vi "Generate_WayPoints_Hopping_CV_AntiDrift.vi"(11 "Input Cluster":T2={"Scan Rate (um/s)"=15.0, "X Start"=15.0, "X End"=15.0, "Y Start"=15.0, "Y End"=15.0, " Z Start"=15.0, "HoppingDistance"=1.0, "V"=15.0, "Z End"=15.0, "Approach Rate Hopping (um/s)"=15.0, "Retrack Rate (um/s)"=15.0, "V 2"=15.0, "Approach Rate (um/s)"=15.0, "V 3"=15.0, "CV Rate / V/s"=15.0, "V 4"=15.0, "V 1"=15.0, "HoldTime1/s"=15.0, "Hold time 2 / s"=15.0, "Hold time 3/ s"=15.0}) -> (0 "output cluster":T1)   [LabVIEW 2023]
uses:
  TypeDefs/WayPointCluster.ctl
  User_Vi/Settings.vi
panel:
  in  "WayPointCluster":T1
  out "Y  P":dbl
  out "X  P":dbl
  out "HoppingDistanceX":dbl
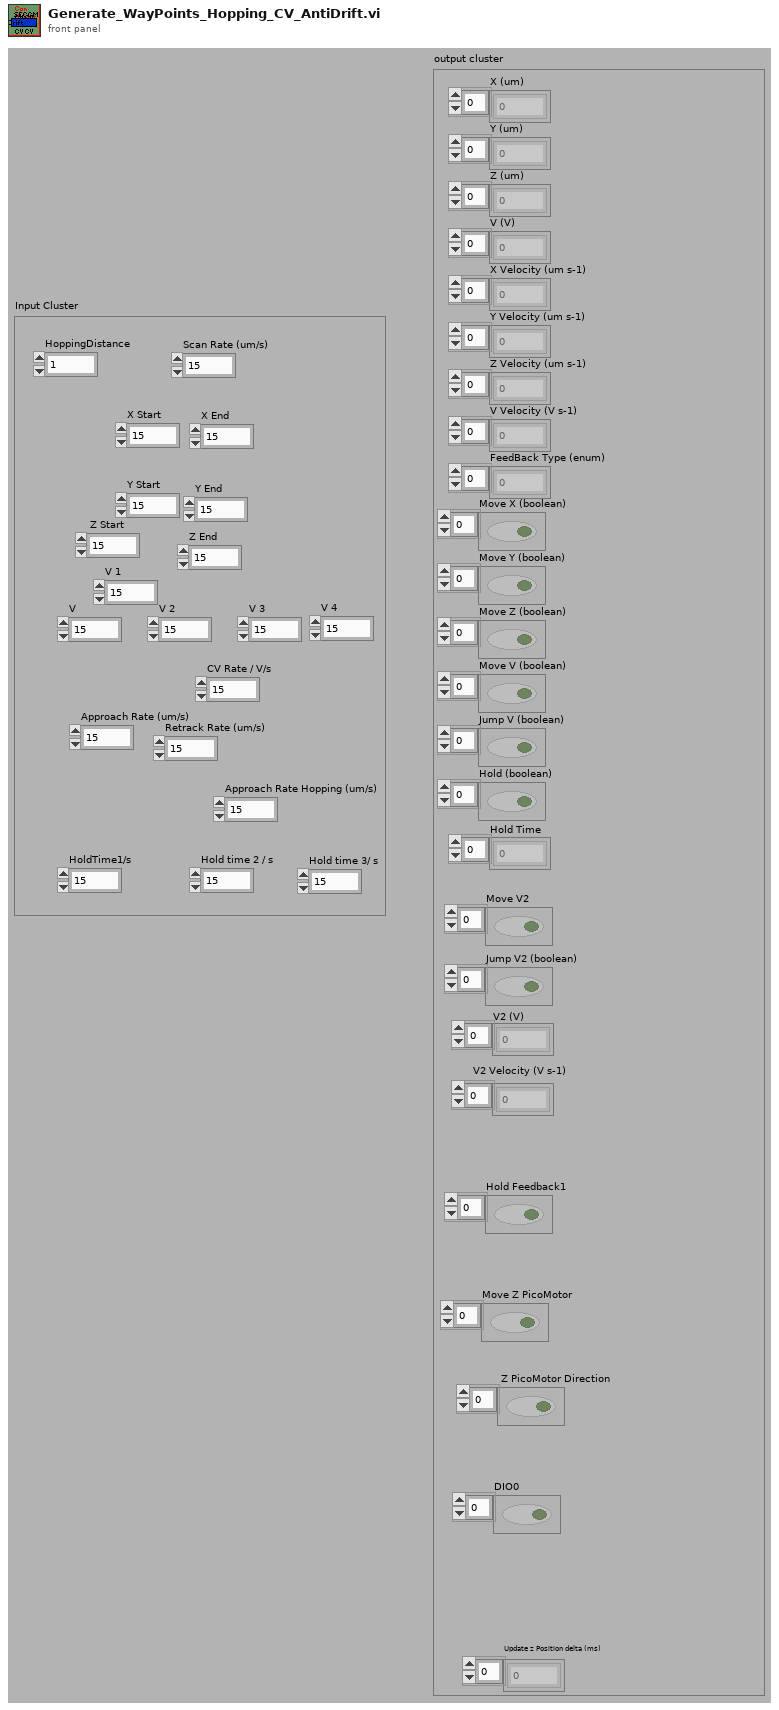
[diagram p1: front panel]
types:
  T1 = typedef "WayPointCluster.ctl" = cluster{"X (um)":dbl[], "Y (um)":dbl[], "Z (um)":dbl[], "V (V)":dbl[], "X Velocity (um s-1)":dbl[], "Y Velocity (um s-1)":dbl[], "Z Velocity (um s-1)":dbl[], "V Velocity (V s-1)":dbl[], "FeedBack Type (enum)":u16[], "Move X (boolean)":bool[], "Move Y (boolean)":bool[], "Move Z (boolean)":bool[], "Move V (boolean)":bool[], "Jump V (boolean)":bool[], "Hold (boolean)":bool[], "Hold Time":u32[], "V2 (V)":dbl[], "Move V2":bool[], "V2 Velocity (V s-1)":dbl[], "Jump V2 (boolean)":bool[], "Update z Position delta (ms)":i16[], "Hold Feedback1":bool[], "Move Z PicoMotor":bool[], " Z PicoMotor Direction":bool[], "DIO0":bool[]}
  T2 = cluster{"Scan Rate (um/s)":dbl, "X Start":dbl, "X End":dbl, "Y Start":dbl, "Y End":dbl, " Z Start":dbl, "HoppingDistance":dbl, "V":dbl, "Z End":dbl, "Approach Rate Hopping (um/s)":dbl, "Retrack Rate (um/s)":dbl, "V 2":dbl, "Approach Rate (um/s)":dbl, "V 3":dbl, "CV Rate / V/s":dbl, "V 4":dbl, "V 1":dbl, "HoldTime1/s":dbl, "Hold time 2 / s":dbl, "Hold time 3/ s":dbl}
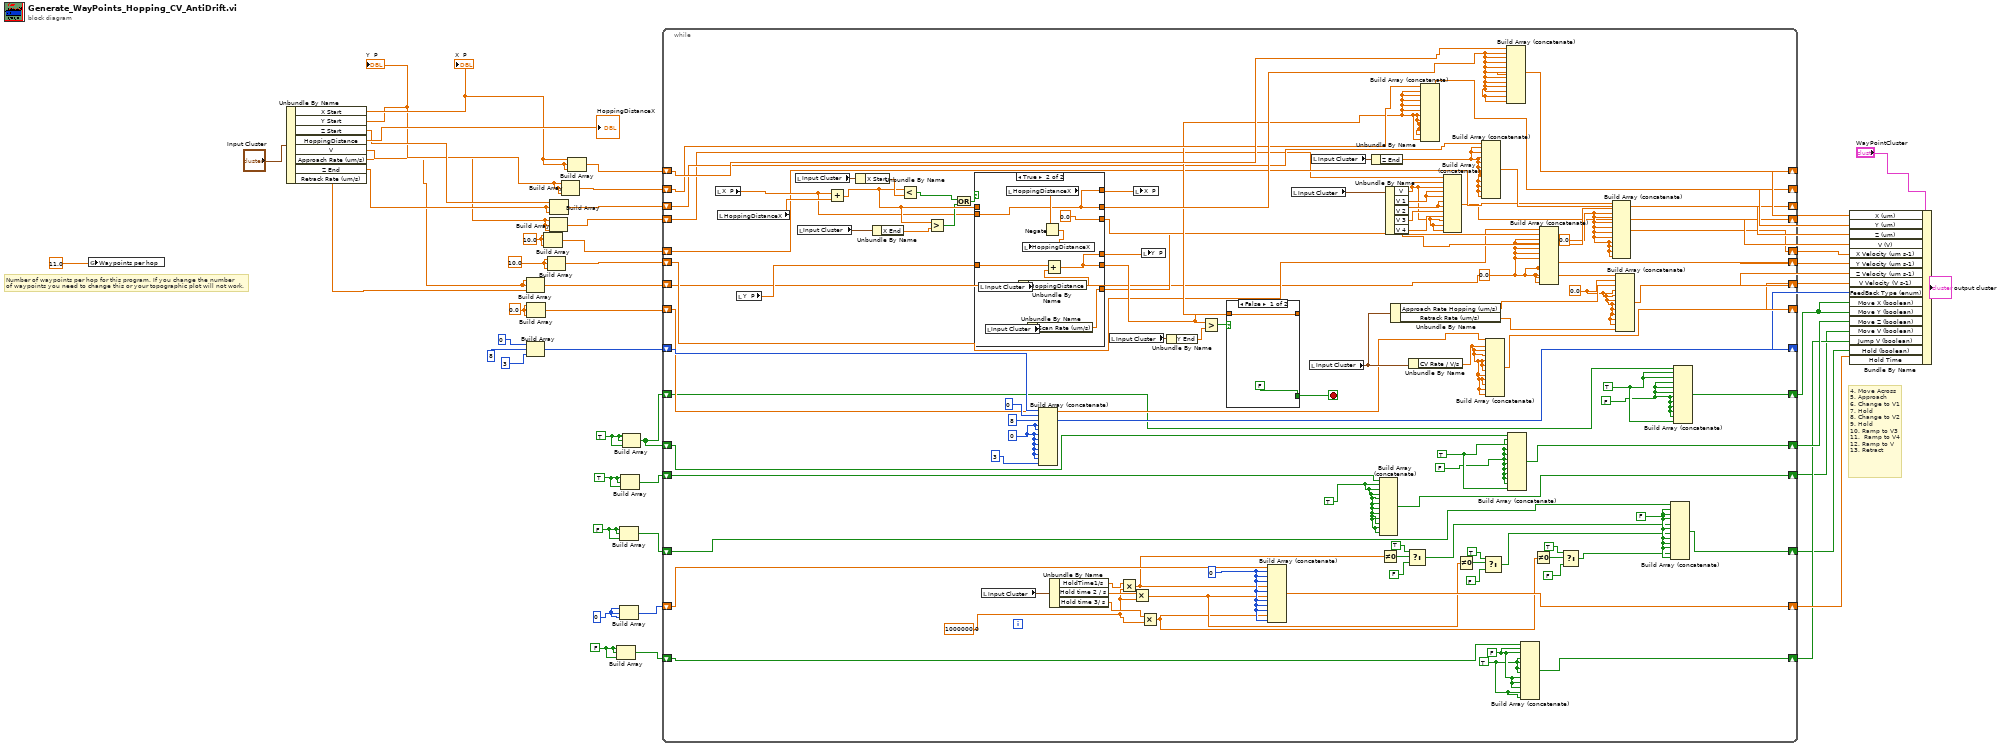
[diagram p0: block diagram]
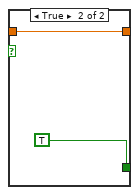
[diagram p2: hidden frame]
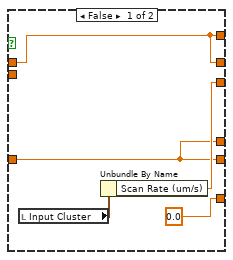
[diagram p3: hidden frame]
diagram:
  w13 = FALSE
  w17 = FALSE
  w16 = u32 0 ("element")
  w15 = TRUE
  w11 = TRUE
  w7 = 10.0 ("element")
  w8 = 10.0 ("element")
  w10 = 0.0 ("element")
  # "Number of waypoints per hop for this program. If you change the number\nof waypoints you need to change this or your topographic plot will not work."
  # "4. Move Across\n5. Approach\n6. Change to V1\n7. Hold\n8. Change to V2\n9. Hold\n10. Ramp to V3\n11.  Ramp to V4\n12. Ramp to V\n13. Retract"
  n1 = global write "Settings.vi" "Waypoints per hop"(11.0) -> ()
  n2 = Unbundle By Name("Input Cluster") -> ("X Start"=w31:dbl, "Y Start"=w30:dbl, "Z Start"=w32:dbl, "HoppingDistance"=→"HoppingDistanceX":dbl, "V"=w28:dbl, "Approach Rate (um/s)"=w9:dbl, "Z End"=w29:dbl, "Retrack Rate (um/s)"=w27:dbl)
  "X  P" <- w31
  "Y  P" <- w30
  n3 = Build Array(w9, w9, w27) -> (w39:dbl[])
  n4 = Build Array(u16 0 ("element"), u16 8 ("element"), u16 3 ("element")) -> (w35:u16[])
  n5 = Build Array(w10, w10, w10) -> (w37:dbl[])
  n6 = Build Array(w7, w7, w7) -> (w42:dbl[])
  n7 = Build Array(w8, w8, w8) -> (w41:dbl[])
  n8 = Build Array(w28, w28, w28) -> (w44:dbl[])
  n9 = Build Array(w32, w29, w29) -> (w46:dbl[])
  n10 = Build Array(w30, w30, w30) -> (w48:dbl[])
  n11 = Build Array(w31, w31, w31) -> (w50:dbl[])
  n12 = Build Array(w17, w17, w17) -> (w21:bool[])
  n13 = Build Array(w13, w13, w13) -> (w12:bool[])
  n14 = Build Array(w16, w16, w16) -> (w24:u32[])
  n15 = Build Array(w15, w15, w15) -> (w19:bool[])
  n16 = Build Array(w11, w11, w11) -> (w3:bool[])
  n17 = while {
    shift-right: [w124] -> w49
    shift-left: w50 -> [w125]
    shift-right: [w121] -> w47
    shift-left: w48 -> [w122]
    shift-right: [w118] -> w45
    shift-left: w46 -> [w119]
    shift-right: [w108] -> w43
    shift-left: w44 -> [w109]
    shift-right: [w102] -> w25
    shift-left: w42 -> [w116]
    shift-right: [w111] -> w40
    shift-left: w41 -> [w112]
    shift-right: [w100] -> w38
    shift-left: w39 -> [w101]
    shift-right: [w95] -> w36
    shift-left: w37 -> [w96]
    shift-right: [w148] -> w34
    shift-left: w35 -> [w149]
    shift-right: [w92] -> w23
    shift-left: w3 -> [w93]
    shift-right: [w58] -> w2
    shift-left: w12 -> [w87]
    shift-right: [w84] -> w22
    shift-left: w24 -> [w85]
    shift-right: [w77] -> w20
    shift-left: w21 -> [w78]
    shift-right: [w89] -> w14
    shift-left: w19 -> [w90]
    shift-right: [w70] -> w4
    shift-left: w3 -> [w69]
    stop <- w136 stop-if-true
    w72 = FALSE
    w73 = TRUE
    w74 = 1000000.0 ("y")
    w75 = TRUE
    w114 = 0.0 ("element")
    w88 = TRUE
    w76 = FALSE
    w79 = u32 0 ("element")
    w86 = FALSE
    w71 = FALSE
    w91 = TRUE
    w127 = u16 0 ("element")
    w110 = 0.0 ("element")
    w98 = 0.0 ("element")
    n18 = local read "X  P"() -> (w135:dbl)
    n19 = local read "HoppingDistanceX"() -> (w150:dbl)
    n20 = local read "Y  P"() -> (w134:dbl)
    n21 = local read "Input Cluster"() -> (w152:T2)
    n22 = local read "Input Cluster"() -> (w151:T2)
    n23 = Add(x=w135, y=w150) -> (x+y=w142:dbl)
    n24 = Unbundle By Name(w152) -> ("X Start"=w145:dbl)
    n25 = Unbundle By Name(w151) -> ("X End"=w143:dbl)
    n26 = Less?(x=w142, y=w145) -> (x < y?=w144:bool)
    n27 = Greater?(x=w142, y=w143) -> (0:w141:bool)
    n28 = Or(x=w144, y=w141) -> (x .or. y?=w140:bool)
    n29 = case shown="True" w140 {
      tunnel: w142 -> [w157 _]
      tunnel: [w157 w163] -> w123
      tunnel: w135 -> [_ w163]
      tunnel: w134 -> [w158 w164]
      tunnel: [w158 w162] -> w133
      tunnel: [w160 0.0] -> w115
      tunnel: [0.0 w165] -> w113
      tunnel: [w158 w162] -> w132
      tunnel: [w157 w163] -> w131
      frame False {
        n30 = local read "Input Cluster"() -> (w161:T2)
        n31 = Unbundle By Name(w161) -> ("Scan Rate (um/s)"=w160:dbl)
      }
      frame True {
        n32 = local read "Input Cluster"() -> (w169:T2)
        n33 = local read "Input Cluster"() -> (w167:T2)
        n34 = local read "HoppingDistanceX"() -> (w171:dbl)
        n35 = Unbundle By Name(w169) -> ("HoppingDistance"=w168:dbl)
        n36 = Unbundle By Name(w167) -> ("Scan Rate (um/s)"=w165:dbl)
        n37 = Negate(x=w171) -> (-x=w170:dbl)
        n38 = local write "HoppingDistanceX"(w170) -> ()
        n39 = Add(x=w164, y=w168) -> (x+y=w162:dbl)
      }
    }
    n40 = local read "Input Cluster"() -> (w83:T2)
    n41 = Build Array (concatenate)(w149, u16 0 ("element"), u16 8 ("element"), w127, w127, w127, w127, w127, w127, w127, w127, u16 3 ("element")) -> (w148:u16[])
    n42 = Unbundle By Name(w83) -> ("HoldTime1/s"=w82:dbl, "Hold time 2 / s"=w81:dbl, "Hold time 3/ s"=w80:dbl)
    n43 = local read "Input Cluster"() -> (w139:T2)
    n44 = Multiply(x=w82, y=w74) -> (x*y=w65:dbl)
    n45 = Multiply(x=w81, y=w74) -> (x*y=w59:dbl)
    n46 = local write "X  P"(w131) -> ()
    n47 = Multiply(x=w80, y=w74) -> (x*y=w54:dbl)
    n48 = local write "Y  P"(w132) -> ()
    n49 = Unbundle By Name(w139) -> ("Y End"=w138:dbl)
    n50 = Greater?(x=w133, y=w138) -> (0:w137:bool)
    n51 = case shown="False" w137 {
      tunnel: w133 -> [w154 w156]
      tunnel: [w154 w156] -> w120
      tunnel: [FALSE TRUE] -> w136
      frame False {
      }
      frame True {
      }
    }
    n52 = Build Array (concatenate)(w85, w79, w79, w79, w65, w79, w59, w79, w79, w79, w54, w79) -> (w84:dbl[])
    n53 = local read "Input Cluster"() -> (w146:T2)
    n54 = local read "Input Cluster"() -> (w128:T2)
    n55 = local read "Input Cluster"() -> (w147:T2)
    n56 = Unbundle By Name(w147) -> ("Z End"=w117:dbl)
    n57 = Build Array (concatenate)(w90, w88, w88, w88, w88, w88, w88, w88, w88, w88, w88, w88) -> (w89:bool[])
    n58 = Not Equal To 0?(x=w65) -> (x != 0?=w68:bool)
    n59 = Unbundle By Name(w146) -> ("V"=w103:dbl, "V 1"=w107:dbl, "V 2"=w106:dbl, "V 3"=w105:dbl, "V 4"=w104:dbl)
    n60 = Unbundle By Name(w128) -> ("Approach Rate Hopping (um/s)"=w99:dbl, "Retrack Rate (um/s)"=w97:dbl)
    n61 = Select(t=TRUE, s=w68, f=FALSE) -> (s? t:f=w64:bool)
    n62 = Unbundle By Name(w128) -> ("CV Rate / V/s"=w94:dbl)
    n63 = Build Array (concatenate)(w122, w120, w120, w120, w120, w120, w120, w120, w120, w120, w120, w120) -> (w121:dbl[])
    n64 = Build Array (concatenate)(w109, w103, w103, w107, w107, w106, w106, w105, w104, w103, w103, w103) -> (w108:dbl[])
    n65 = Not Equal To 0?(x=w59) -> (x != 0?=w63:bool)
    n66 = Build Array (concatenate)(w119, w117, w117, w117, w117, w117, w117, w117, w117, w117, w117, w117) -> (w118:dbl[])
    n67 = Select(t=TRUE, s=w63, f=FALSE) -> (s? t:f=w60:bool)
    n68 = Build Array (concatenate)(w96, w94, w94, w94, w94, w94, w94, w94, w94, w94, w94, w94) -> (w95:dbl[])
    n69 = Build Array (concatenate)(w125, w123, w123, w123, w123, w123, w123, w123, w123, w123, w123, w123) -> (w124:dbl[])
    n70 = Build Array (concatenate)(w93, w71, w91, w71, w71, w71, w71, w71, w71, w71, w71, w91) -> (w92:bool[])
    n71 = Build Array (concatenate)(w78, w76, w76, w75, w75, w75, w75, w76, w76, w76, w75, w75) -> (w77:bool[])
    n72 = Not Equal To 0?(x=w54) -> (x != 0?=w56:bool)
    n73 = Build Array (concatenate)(w112, w113, w110, w110, w110, w110, w110, w110, w110, w110, w110, w110) -> (w111:dbl[])
    n74 = Select(t=TRUE, s=w56, f=FALSE) -> (s? t:f=w53:bool)
    n75 = Build Array (concatenate)(w116, w115, w114, w114, w114, w114, w114, w114, w114, w114, w114, w114) -> (w102:dbl[])
    n76 = Build Array (concatenate)(w101, w98, w99, w98, w98, w98, w98, w98, w98, w98, w98, w97) -> (w100:dbl[])
    n77 = Build Array (concatenate)(w87, w86, w86, w86, w64, w86, w60, w86, w86, w86, w53, w86) -> (w58:bool[])
    n78 = Build Array (concatenate)(w69, w73, w73, w72, w72, w72, w72, w72, w72, w72, w72, w73) -> (w70:bool[])
  }
  n79 = Bundle By Name(cluster="WayPointCluster", "X (um)"=w49, "Y (um)"=w47, "Z (um)"=w45, "V (V)"=w43, "X Velocity (um s-1)"=w25, "Y Velocity (um s-1)"=w40, "Z Velocity (um s-1)"=w38, "V Velocity (V s-1)"=w36, "FeedBack Type (enum)"=w34, "Move X (boolean)"=w4, "Move Y (boolean)"=w4, "Move Z (boolean)"=w23, "Move V (boolean)"=w14, "Jump V (boolean)"=w20, "Hold (boolean)"=w2, "Hold Time"=w22) -> (→"output cluster":T1)
